vi "Up.vi"(0 "Enable":bool=TRUE, 5 "error in (no error)":errorcluster) -> (15 "Valve Opening":dbl caption="Степень открытия клапана Valve 1" format="%#g", 16 "Pump power":dbl caption="Мощность насоса" format="%#g", 17 "Filling tim":dbl caption="Время заполнения" format="%#g", 18 "Сonfirm":bool caption="OK", 19 "error out":errorcluster)   [LabVIEW 2014]
doc: "Displays a standard dialog box that prompts users to enter information, such as a user name and password.\n--------------------\n\nThis Express VI is configured as follows:\n\nMessage to Display to the User:Срабатывание сигнализатора верхнего уровня! Укажите время в секундах для снижения уровня жидкости в нижней ёмкости!\nThe inputs are: \nNumber: Время заполнения\nNumber: Мощность насоса\nNumber: Степень открытия клапана Valve 1"
panel:
  in  "Valve Opening":dbl caption="Степень открытия клапана Valve 1" min=0.0 max=100.0 step=0.5 format="%#g"
  in  "Pump power":dbl caption="Мощность насоса" min=0.0 max=5.0 step=1.0 format="%#g"
  in  "Filling time":dbl caption="Время заполнения" min=0.0 max=300.0 step=0.5 format="%#g"
  out "String":string="Срабатывание сигнализатора верхнего уровня! Укажите время в секундах для снижения уровня жидкости в нижней ёмкости!"
  in  "Cancel":bool
  in  "OK2":bool
  in  "OK1":bool
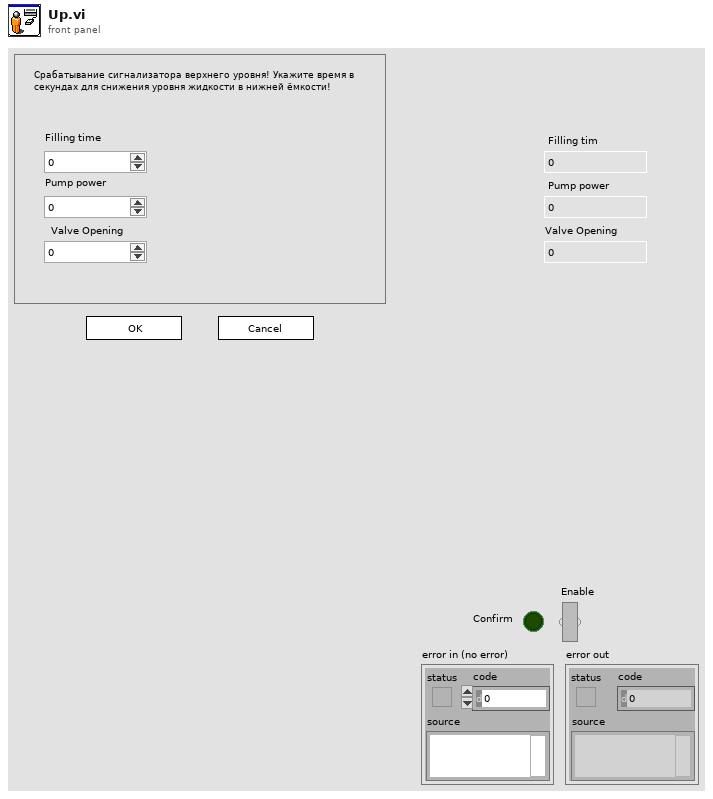
[diagram p1: front panel]
types:
  T1 = cluster{"Input Name":string, "Input Data Type":i32}[]
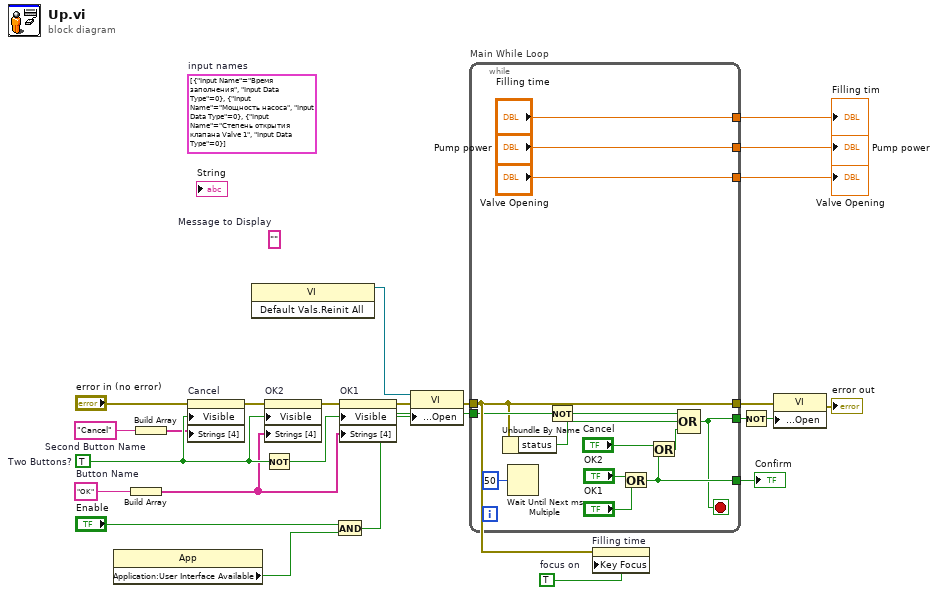
[diagram p0: block diagram]
diagram:
  w3 = TRUE  # focus on
  (unwired) T1 [{"Input Name"="Время заполнения", "Input Data Type"=0}, {"Input Name"="Мощность насоса", "Input Data Type"=0}, {"Input Name"="Степень открытия клапана Valve 1", "Input Data Type"=0}]  # input names
  w16 = "Cancel"  # Second Button Name
  w14 = "OK"  # Button Name
  (unwired) ""  # Message to Display
  w24 = TRUE  # Two Buttons?
  n1 = property class="App"() -> ("Application:User Interface Available"=w6:bool)  [unwired: 2 in, 2 out]
  n2 = Build Array(w14) -> (w15:string[])
  n3 = Build Array(w16) -> (w17:string[])
  n4 = property on="Cancel" class="Bool"(error in="error in (no error)", "Visible"=w24, "Strings [4]"=w17) -> (error out=w21:errorcluster)  [unwired: 1 in, 1 out]
  n5 = invoke class="VI" method="Default Vals.Reinit All"() -> (reference out=w5:refnum<vi>)  [unwired: 3 in, 2 out]
  n6 = Not(x=w24) -> (.not. x?=w22:bool)
  n7 = property on="OK2" class="Bool"(error in=w21, "Visible"=w24, "Strings [4]"=w15) -> (error out=w20:errorcluster)  [unwired: 1 in, 1 out]
  n8 = And(x="Enable", y=w6) -> (x .and. y?=w7:bool)
  n9 = property on="OK1" class="Bool"(error in=w20, "Visible"=w22, "Strings [4]"=w15) -> (error out=w13:errorcluster)  [unwired: 1 in, 1 out]
  n10 = property class="VI"(reference=w5, error in=w13, "Front Panel Window:Open"=w7) -> (error out=w12:errorcluster)  [unwired: 1 out]
  n11 = while "Main While Loop" {
    tunnel: [w35] -> w23
    tunnel: w7 -> [w33]
    tunnel: [w31] -> w18
    tunnel: w12 -> [w30]
    tunnel: [w30] -> w10
    tunnel: ["Filling time"] -> w4
    tunnel: ["Pump power"] -> w2
    tunnel: ["Valve Opening"] -> w1
    stop <- w31 stop-if-true
    n12 = Unbundle By Name(w30) -> ("status"=w28:bool)
    n13 = Wait Until Next ms Multiple(millisecond multiple=u32 50) -> ()  [unwired: 1 out]
    n14 = Not(x=w33) -> (.not. x?=w32:bool)
    n15 = Or(x="OK2", y="OK1") -> (x .or. y?=w35:bool)
    n16 = Or(x="Cancel", y=w35) -> (x .or. y?=w29:bool)
    n17 = Compound Arithmetic op=OR(w32, w28, w29) -> (w31:bool)
  }
  "Сonfirm" <- w23
  "Filling tim" <- w4
  "Pump power" <- w2
  "Valve Opening" <- w1
  n18 = property on="Filling time" class="DigNum (strict)"(error in=w12, "Key Focus"=w3) -> ()  [unwired: 1 in, 2 out]
  n19 = Not(x=w18) -> (.not. x?=w19:bool)
  n20 = property class="VI"(error in=w10, "Front Panel Window:Open"=w19) -> (error out=→"error out":errorcluster)  [unwired: 1 in, 1 out]
